vi "Score Display - Display Image (LV).vi"(2 "image data":T1, 3 "Picture Reference":refnum<vi>) -> ()   [LabVIEW 2013]
uses:
  <vilib>/picture/picture.llb/imagedata.ctl
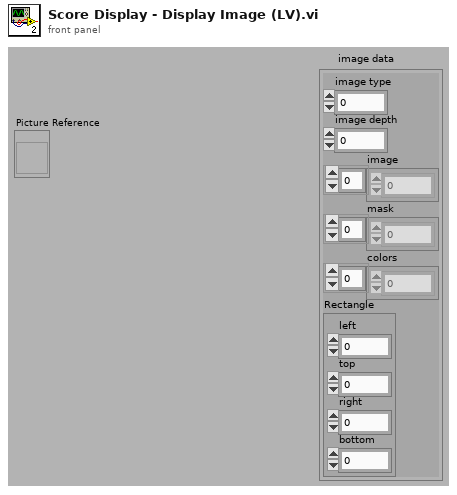
[diagram p1: front panel]
types:
  T1 = typedef "imagedata.ctl" = cluster{"image type":i32, "image depth":i32, "image":u8[], "mask":u8[], "colors":u32[], "Rectangle":cluster{"left":i16, "top":i16, "right":i16, "bottom":i16}}
  T2 = cluster{"left":i16, "top":i16, "right":i16, "bottom":i16}
  T3 = typedef "LVBoundsTypeDef.ctl" = cluster{"Width":u32, "Height":u32}
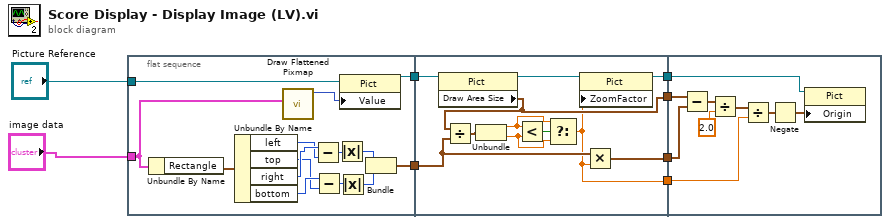
[diagram p0: block diagram]
diagram:
  n1 = flat-sequence {
    tunnel: [w13] -> w8
    tunnel: [w10] -> w7
    tunnel: "Picture Reference" -> [w12]
    tunnel: "image data" -> [w9]
    tunnel: w8 -> [w28]
    tunnel: [w27] -> w6
    tunnel: [w25] -> w5
    tunnel: [w24] -> w4
    tunnel: w7 -> [w26]
    tunnel: [w22] -> w3
    tunnel: w6 -> [w40]
    tunnel: w5 -> [w41]
    tunnel: w4 -> [w36]
    tunnel: w3 -> [w33]
    frame #0 {
      n2 = Unbundle By Name(w9) -> ("Rectangle"=w21:T2)
      n3 = Unbundle By Name(w21) -> ("left"=w19:i16, "top"=w17:i16, "right"=w20:i16, "bottom"=w18:i16)
      n4 = call <vilib>:"Draw Flattened Pixmap.vi"("image data"=w9) -> ("new picture"=w11:picture)  [unwired: 1 in, 7 out]
      n5 = Subtract(x=w20, y=w19) -> (x-y=w15:i16)
      n6 = Subtract(x=w18, y=w17) -> (x-y=w16:i16)
      n7 = Absolute Value(x=w15) -> ()  [unwired: 1 out]
      n8 = Absolute Value(x=w16) -> (abs(x)=w14:i16)
      n9 = property class="Pict"(reference=w12, "Value"=w11) -> (reference out=w10:refnum<vi>)  [unwired: 1 in, 1 out]
      n10 = Bundle(w15, w14) -> (w13:cluster{i16, i16})  [unwired: 1 out]
    }
    frame #1 {
      n11 = property class="Pict"(reference=w26) -> (reference out=w23:refnum<vi>, "Draw Area Size"=w25:T3)  [unwired: 1 in, 1 out]
      n12 = Divide(x=w25, y=w28) -> (x/y=w32:cluster{dbl, dbl})
      n13 = Unbundle(w32) -> (w30:dbl, w29:dbl)
      n14 = Less?(x=w30, y=w29) -> (x < y?=w31:bool)
      n15 = Select(t=w30, s=w31, f=w29) -> (s? t:f=w24:dbl)
      n16 = property class="Pict"(reference=w23, "ZoomFactor"=w24) -> (reference out=w22:refnum<vi>)  [unwired: 1 in, 1 out]
      n17 = Multiply(x=w28, y=w24) -> (x*y=w27:cluster{dbl, dbl})
    }
    frame #2 {
      n18 = Subtract(x=w41, y=w40) -> (x-y=w38:cluster{dbl, dbl})
      n19 = Divide(x=w38, y=2.0) -> (x/y=w37:cluster{dbl, dbl})
      n20 = Divide(x=w37, y=w36) -> (x/y=w35:cluster{dbl, dbl})
      n21 = Negate(x=w35) -> (-x=w34:cluster{dbl, dbl})
      n22 = property class="Pict"(reference=w33, "Origin"=w34) -> ()  [unwired: 1 in, 2 out]
    }
  }
